vi "Compute Square-Gated Discrete Calibration Phasor & jw.vi"(6 "Gate Width (W)":dbl[unit], 8 "Laser Period (T)":dbl[unit], 9 "Calibration Lifetime (tau)":dbl[unit], 10 "# Gates (N)":dbl, 11 "Harmonic frequency (f)":dbl[unit]) -> (2 "Z_N[W](tau)":cdb, 3 "i 2 pi f (GHz)":cdb)   [LabVIEW 2019]
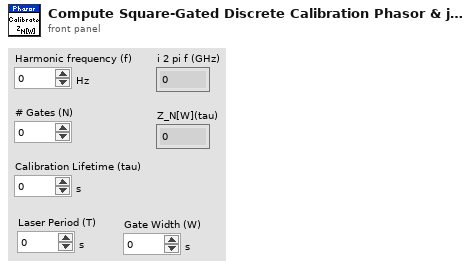
[diagram p1: front panel]
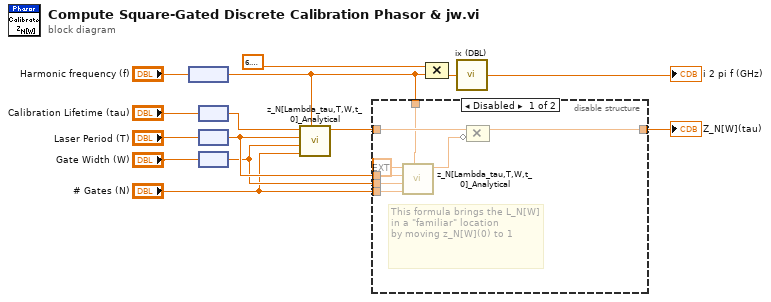
[diagram p0: block diagram]
diagram:
  n1 = node("Harmonic frequency (f)") -> (w1:dbl)
  n2 = node("Calibration Lifetime (tau)") -> (w6:dbl)
  n3 = node("Laser Period (T)") -> (w5:dbl)
  n4 = node("Gate Width (W)") -> (w4:dbl)
  n5 = call "z_N[Lambda_tau,T,W,t_0]_Analytical.vi"("Harmonic f"=w1, "N"="# Gates (N)", "W"=w4, "T"=w5, "tau"=w6) -> ("z_n,N,W(tau)"=w7:cxt)  [unwired: 6 in]
  n6 = disable-structure shown="Disabled" {
    disable-tunnel: w7 -> [w22 w23]
    disable-tunnel: w5 -> [w21 _]
    disable-tunnel: w4 -> [w20 _]
    disable-tunnel: "# Gates (N)" -> [w19 _]
    disable-tunnel: [w17 w23] -> w2
    disable-tunnel: w1 -> [w15 _]
    frame Disabled {
      # "This formula brings the L_N[W] in a \"familiar\" location\nby moving z_N[W](0) to 1"
      n7 = call "z_N[Lambda_tau,T,W,t_0]_Analytical.vi"("Harmonic f"=w15, "N"=w19, "W"=w20, "T"=w21, "tau"=ext 0.0) -> ("z_n,N,W(tau)"=w16:cxt)  [unwired: 6 in]
      n8 = Compound Arithmetic op=MULTIPLY(w22, invert w16) -> (w17:cxt)
    }
    frame Enabled {
    }
  }
  "Z_N[W](tau)" <- w2
  n9 = Compound Arithmetic op=MULTIPLY(6.283185307179586, w1) -> (w14:dbl)
  n10 = call "ix (DBL).vi"("x (1)"=w14) -> ("i.(x)"=→"i 2 pi f (GHz)":cdb)
